vi "GetAppRefInArray.vi"() -> (0 "error out":errorcluster, 1 "Array":refnum<vi>[](array[refnum]))   [LabVIEW 2012]
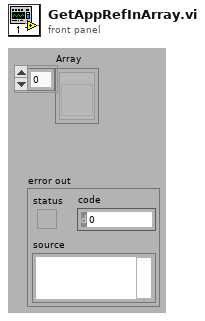
[diagram p1: front panel]
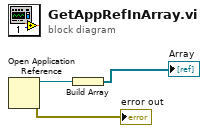
[diagram p0: block diagram]
diagram:
  n1 = Open Application Reference() -> (0:→"error out":errorcluster, 3:w2:refnum<vi>)  [unwired: 1 in, 3 out]
  n2 = Build Array(w2) -> (→"Array":refnum<vi>[])
